vi "Read Test Parameters.vi"(11 "TestMonitor in":refnum<class "TestMonitor.lvclass">) -> (2 "Test Parameters":T1 {"Max records per file" min=100 max=1000000; "Cycle profile"."Pause After" min=1.0 max=600.0 format="%.1f"; "Cycle profile"."Force Setpoint" min=-556.0 max=556.0 format="%.1f"; "Number of cycles for complete test" min=1}, 3 "TestMonitor out":refnum<class "TestMonitor.lvclass">)   [LabVIEW 2013, in "TestMonitor.lvclass"]
uses:
  TestMonitor.lvclass
  Configuration/Test Parameters.ctl
  Configuration/CycleProfileConfig.ctl
  TestMonitor.lvclass/TestMonitor.ctl
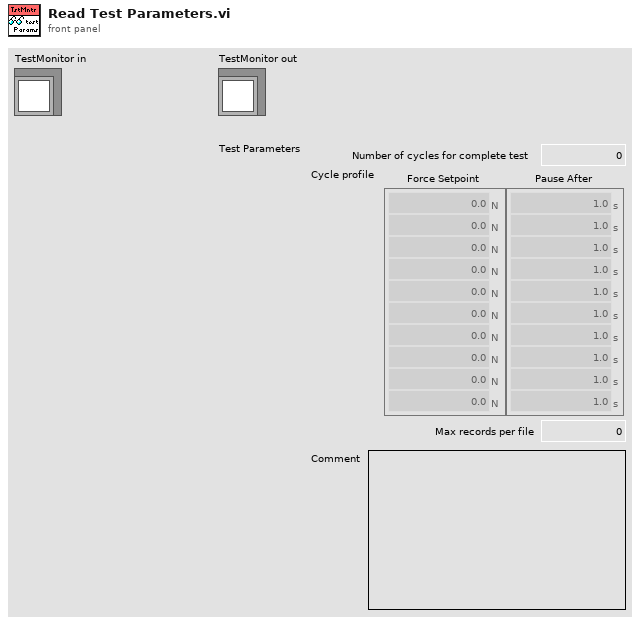
[diagram p1: front panel]
types:
  T1 = typedef "Test Parameters.ctl" = cluster{"Number of cycles for complete test":u32, "Cycle profile":T2, "Max records per file":u32, "Comment":string}
  T2 = typedef "CycleProfileConfig.ctl" = cluster{"Force Setpoint":dbl[unit][], "Pause After":dbl[unit][]}
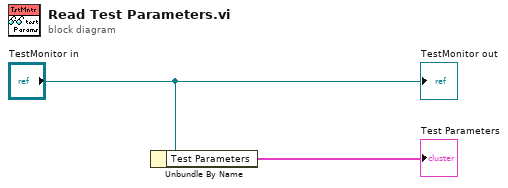
[diagram p0: block diagram]
diagram:
  n1 = Unbundle By Name("TestMonitor in") -> ("Test Parameters"=→"Test Parameters":T1)
  "TestMonitor out" <- "TestMonitor in"
